vi "Write ColorDaysOfWeekBackground.vi"(8 "error in (no error)":errorcluster, 10 "ColorDaysOfWeekBackground":u32(colorbox), 11 "Calendar in":refnum<class "Calendar.lvclass">) -> (0 "error out":errorcluster, 3 "Calendar out":refnum<class "Calendar.lvclass">)   [LabVIEW 2015, in "Calendar.lvclass"]
uses:
  Calendar.lvclass
  Calendar.lvclass/Calendar.ctl
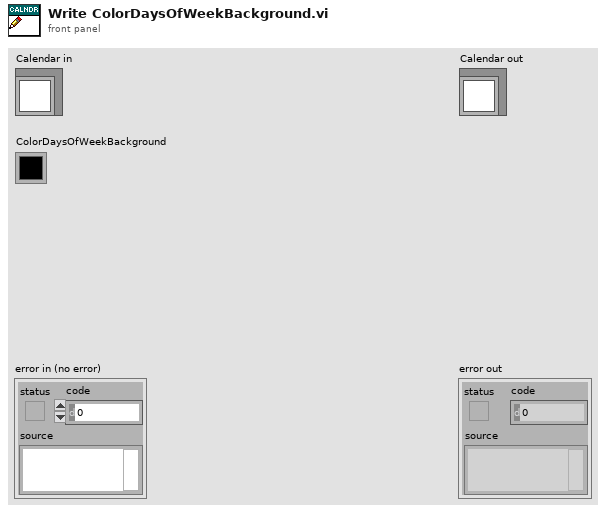
[diagram p1: front panel]
types:
  T1 = typedef "Calendar.lvclass/State Data.ctl" = cluster{"Current Date":timestamp, "First Day of Week":T2, "Color":cluster{"Selector Background":u32, "Selector Text":u32, "Days of Week Background":u32, "Days of Week Text":u32, "Calendar Background":u32, "Calendar Text":u32, "Calendar Selection Background":u32, "Calendar Selection Text":u32}, "Visible":cluster{"Today Selector Visible":bool, "Month-Year Selector Visible":bool}}
  T2 = typedef "Calendar.lvclass/DaysOfWeek.ctl" = enum16{"Sunday", "Monday", "Tuesday", "Wednesday", "Thursday", "Friday", "Saturday"}
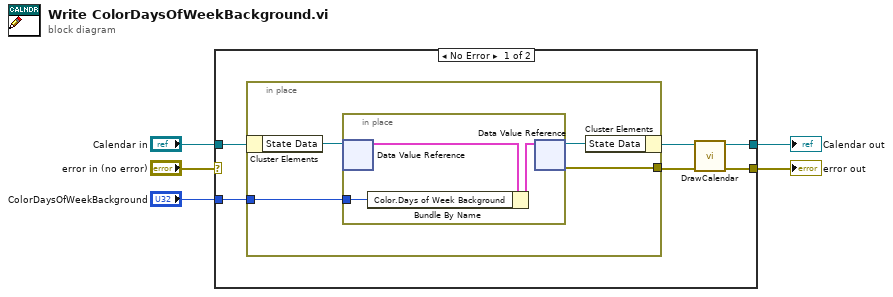
[diagram p0: block diagram]
diagram:
  n1 = case shown="No Error" "error in (no error)" {
    selector: "error in (no error)" -> [_ w20]
    tunnel: [w8 w20] -> w4
    tunnel: [w7 w19] -> w2
    tunnel: "Calendar in" -> [w11 w19]
    tunnel: "ColorDaysOfWeekBackground" -> [w6 _]
    frame No Error {
      n2 = in-place {
        in-place-border: [w13] -> w9
        in-place-border: w6 -> [w12]
        n3 = in-place-cluster #1(w11) -> ("State Data"=w15:refnum<data-value>)
        n4 = in-place {
          in-place-border: w12 -> [w16]
          n5 = in-place-dvr #2(w15) -> (w18:T1)  [unwired: 1 out]
          n6 = Bundle By Name(cluster=w18, "Color.Days of Week Background"=w16) -> (w17:T1)
          n7 = in-place-dvr #2(w17) -> (w14:refnum<data-value>, w13:errorcluster)
        }
        n8 = in-place-cluster #1("State Data"=w14) -> (w10:refnum<class "Calendar.lvclass">)
      }
      n9 = call "DrawCalendar.vi"("error in (no error)"=w9, "Calendar in"=w10) -> ("error out"=w8:errorcluster, "Calendar out"=w7:refnum<class "Calendar.lvclass">)  [unwired: 8 in]
    }
    frame Error {
    }
  }
  "error out" <- w4
  "Calendar out" <- w2
